vi "ODOR_BLASTER_V22.3 Final.vi"() -> ()   [LabVIEW 2022 SP3]
uses:
  <vilib>/Utility/error.llb/DialogType.ctl
  <vilib>/DAQmx/read.llb/DAQmx Read (Analog Wfm 1Chan NSamp).vi
  <vilib>/DAQmx/write.llb/DAQmx Write (Digital 1D Bool NChan 1Samp 1Line).vi
  <vilib>/gmath/statdist.llb/Random Permutation.vi
  <vilib>/DAQmx/create/channels.llb/DAQmx Create Channel (AI-Voltage-Basic).vi
  <vilib>/DAQmx/configure/timing.llb/DAQmx Timing (Sample Clock).vi
  <vilib>/DAQmx/miscellaneous.llb/DAQmx Fill In Error Info.vi
  <vilib>/Waveform/WDTOps.llb/WDT Append Waveforms DBL.vi
  <vilib>/Waveform/WDTFileIO.llb/Export Waveform To Spreadsheet File.vi
  <vilib>/gmath/NI_Gmath.lvlib
panel:
  out "Elapsed Time (s)":dbl
  out "source out 2":string
  out "error out 2":errorcluster
  out "Waveform Chart 2":waveform(dbl)(graph)
  out "source out":string
  out "error out":errorcluster
  out "RECORDING TIME (s)":dbl
  out "Waveform Chart":waveform(dbl)(graph)
  in  "How long recording lasts (s)":u32=4 caption="Time Target (s)"
  out "Device Running":bool
  in  "Time Between Loops (s)":i32=1
  in  "Presentation mode":u8(ring) items=["Sequential", "Random", "Simultaneous"]
  in  "Initial Delay (s)":u32=10
  out "Coming up next":bool[](array[boolean])
  in  "manual trigger":bool
  in  "Number of Puffs per trial":i32=1
  out "Puffing":bool
  in  "Puff Duration (s)":u32=2000
  in  "Valves to use":bool[](array[boolean])
  # "1"
  # "2"
  # "3"
  # "4"
  # "5"
  # "6"
  # "7"
  # "8"
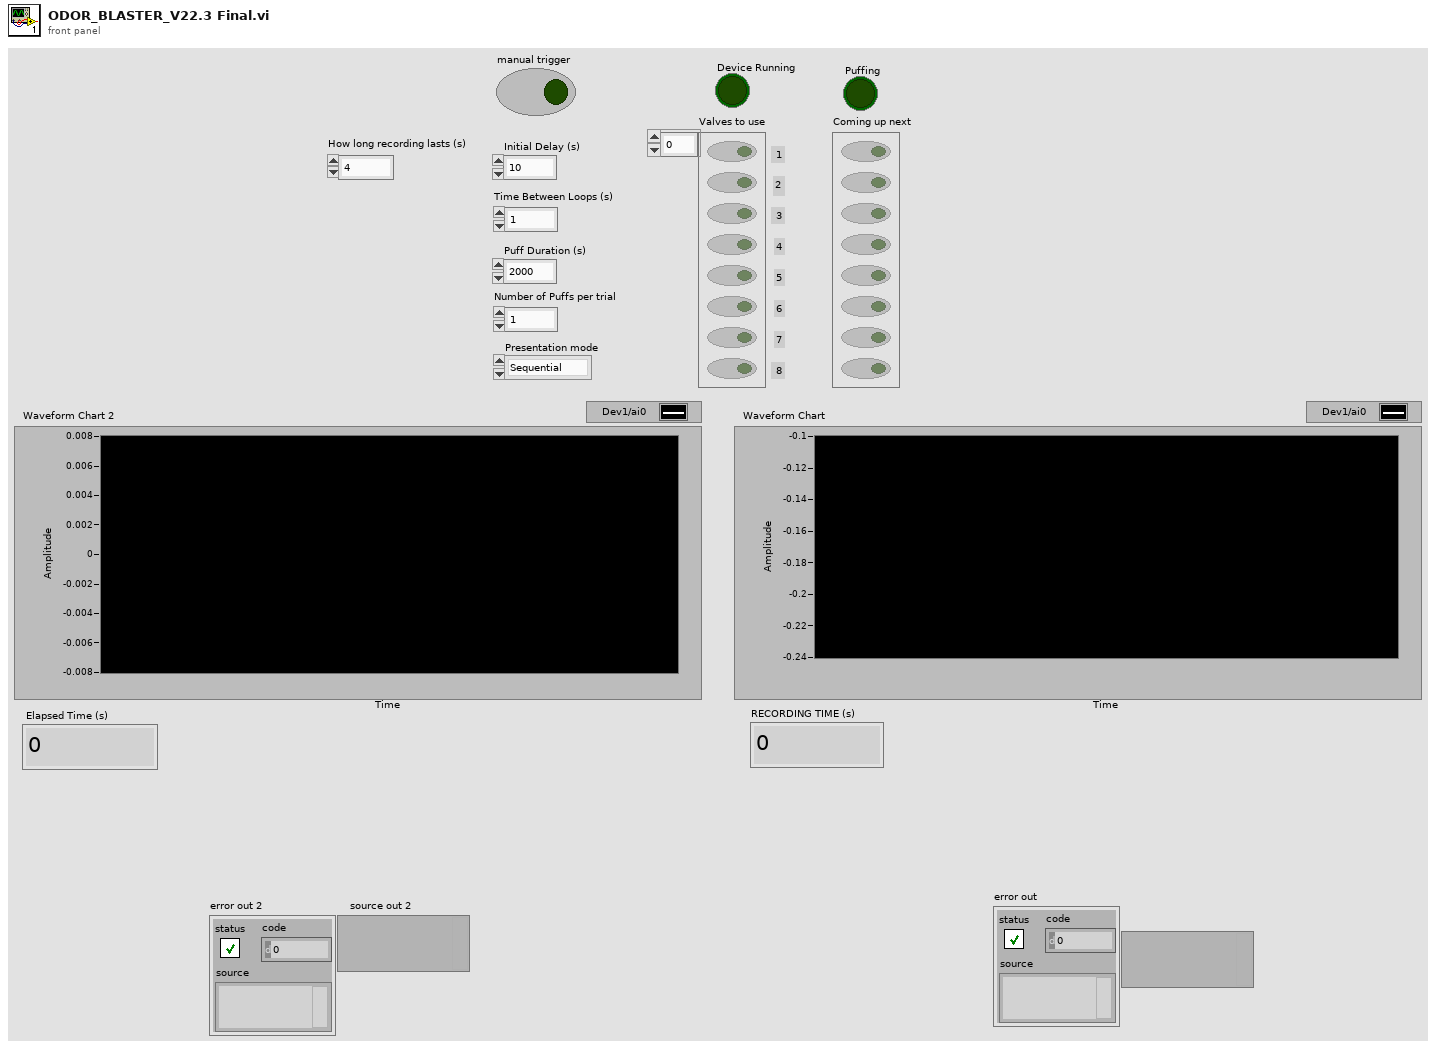
[diagram p1: front panel]
types:
  T1 = typedef "DialogType.ctl" = u16
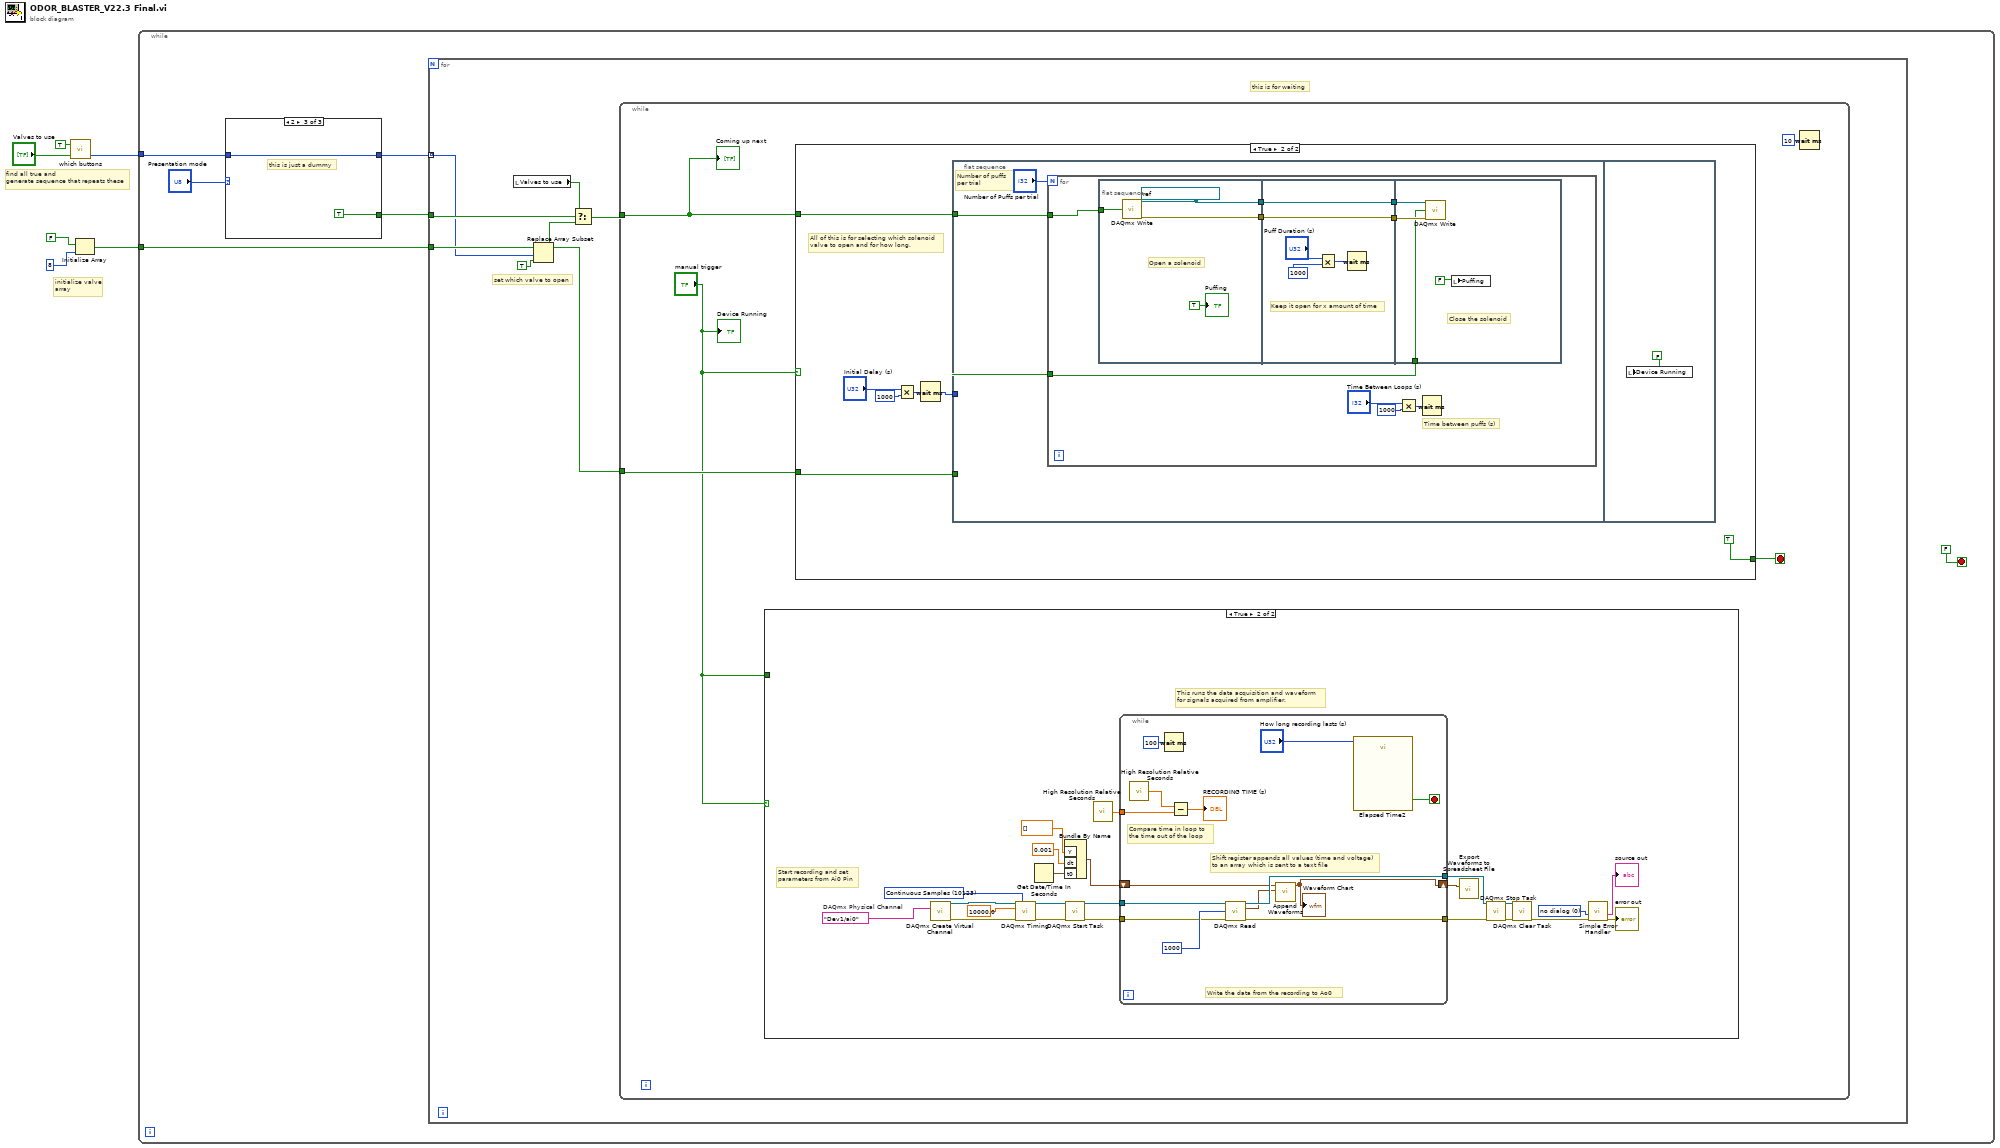
[diagram p0: block diagram]
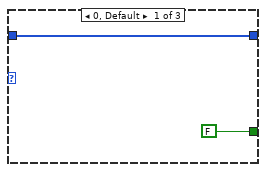
[diagram p2: hidden frame]
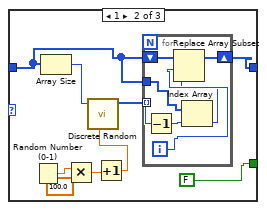
[diagram p3: hidden frame]
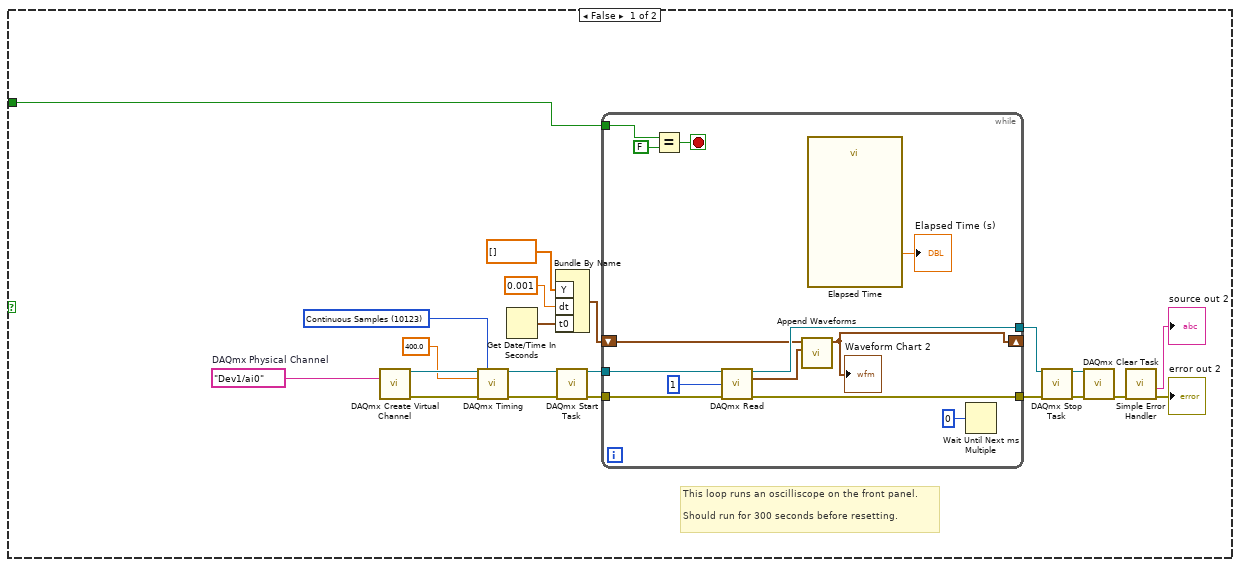
[diagram p4: hidden frame]
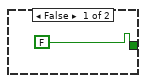
[diagram p5: hidden frame]
diagram:
  # "initialize valve\narray"
  # "find all true and\ngenerate sequence that repeats these"
  n1 = call "which buttons.vi"("boolean array"="Valves to use", "true/false"=TRUE) -> ("indexes of matching booleans"=w4:i32[])  [unwired: 1 in]
  n2 = Initialize Array(FALSE, 8 ("dimension size")) -> (w1:bool[])
  n3 = while {
    tunnel: w4 -> [w10]
    tunnel: w1 -> [w11]
    stop <- FALSE stop-if-true
    n4 = case shown="2" "Presentation mode" {
      tunnel: w10 -> [w14 w21 w32]
      tunnel: [w14 w20 w32] -> w7
      tunnel: [FALSE FALSE TRUE] -> w8
      frame 0, Default {
      }
      frame 1 {
        n5 = Random Number (0-1)() -> (number: 0 to 1=w19:dbl)
        n6 = Array Size(array=w21) -> (size(s)=w23:i32)
        n7 = Multiply(x=w19, y=100.0) -> (x*y=w17:dbl)
        n8 = Increment(x=w17) -> (x+1=w16:dbl)
        n9 = call-poly <vilib>:"Discrete Random.vi"("seed"=w16, "N"=w23) -> ("random permutation"=w22:i32[])  [unwired: 8 in, 1 out]
        n10 = for {
          tunnel: w22 -> [w30] mode=indexing
          shift-right: [w27] -> w20
          shift-left: w21 -> [w28]
          tunnel: w21 -> [w25]
          i -> [w26]
          n11 = Decrement(x=w30) -> (x-1=w29:i32)
          n12 = Index Array(array=w25, index=w29) -> (element=w24:i32)
          n13 = Replace Array Subset(array=w28, new element=w24, index=w26) -> (w27:i32[])
        }
      }
      frame 2 {
        # "this is just a dummy"
      }
    }
    n14 = for {
      tunnel: w11 -> [w37]
      tunnel: w8 -> [w38]
      tunnel: w7 -> [w33] mode=indexing
      # "set which valve to open"
      # "this is for waiting"
      n15 = local read "Valves to use"() -> (w36:bool[])
      n16 = Replace Array Subset(array=w37, new element=TRUE ("new element/subarray"), index=w33) -> (w35:bool[])
      n17 = Select(t=w36, s=w38, f=w35) -> (s? t:f=w34:bool[])
      n18 = while {
        tunnel: w34 -> [w43]
        tunnel: w37 -> [w42]
        stop <- w40 stop-if-true
        n19 = case shown="True" "manual trigger" {
          tunnel: "manual trigger" -> [w45 _]
          frame False {
            w50 = tag "Dev1/ai0"  # DAQmx Physical Channel
            w49 = 10123 items=["Finite Samples"=10178, "Continuous Samples"=10123, "Hardware Timed Single Point"=12522] ("sample mode")
            # "This loop runs an oscilliscope on the front panel.\n\nShould run for 300 seconds before resetting."
            n20 = call-poly <vilib>:"DAQmx Create Virtual Channel.vi"("physical channels"=w50) -> ("task out"=w52:refnum<k21>, "error out"=w51:errorcluster)  [unwired: 13 in]
            n21 = call-poly <vilib>:"DAQmx Timing.vi"("task/channels in"=w52, "sample mode"=w49, "rate"=400.0, "error in"=w51) -> ("task out"=w59:refnum<k21>, "error out"=w60:errorcluster)  [unwired: 10 in]
            n22 = Get Date/Time In Seconds() -> (seconds since 1Jan1904=w58:timestamp)
            n23 = Bundle By Name("Y"=dbl[] [], "dt"=0.001, "t0"=w58) -> (w57:waveform(dbl))  [unwired: 1 in]
            n24 = call <vilib>:"DAQmx Start Task.vi"("task/channels in"=w59, "error in"=w60) -> ("task out"=w61:refnum<k21>, "error out"=w62:errorcluster)  [unwired: 12 in]
            n25 = while {
              tunnel: [w78] -> w53
              tunnel: [w77] -> w54
              tunnel: w61 -> [w74]
              tunnel: w62 -> [w73]
              shift-right: [w70] -> _
              shift-left: w57 -> [w71]
              tunnel: w45 -> [w68]
              stop <- w67 stop-if-true
              n26 = Equal?(x=w68, y=FALSE) -> (x = y?=w67:bool)
              n27 = call-poly <vilib>:"DAQmx Read.vi"("task/channels in"=w74, "number of samples per channel"=1, "error in"=w73) -> ("task out"=w78:refnum<k21>, "data"=w72:waveform(dbl), "error out"=w77:errorcluster)  [unwired: 10 in]
              n28 = call-poly <vilib>:"Append Waveforms.vi"("waveform B"=w72, "waveform A"=w71) -> ("waveform out"=w70:waveform(dbl))  [unwired: 8 in, 1 out]
              "Waveform Chart 2" <- w70
              n29 = call "Elapsed Time"() -> ("Elapsed Time (s)"=→"Elapsed Time (s)":dbl)  [unwired: 12 in, 7 out]
              n30 = Wait Until Next ms Multiple(millisecond multiple=u32 0) -> ()  [unwired: 1 out]
            }
            n31 = call <vilib>:"DAQmx Stop Task.vi"("task/channels in"=w53, "error in"=w54) -> ("task out"=w55:refnum<k21>, "error out"=w56:errorcluster)  [unwired: 12 in]
            n32 = call <vilib>:"DAQmx Clear Task.vi"("task in"=w55, "error in"=w56) -> ("error out"=w63:errorcluster)  [unwired: 13 in]
            n33 = call <vilib>:"Simple Error Handler.vi"("error in (no error)"=w63) -> ("source out"=→"source out 2":string, "error out"=→"error out 2":errorcluster)  [unwired: 4 in, 3 out]
          }
          frame True {
            w81 = T1 0 items=["no dialog", "OK message", "continue or stop message", "OK message + warnings", "continue/stop + warnings"] ("type of dialog (OK msg:1)")
            w97 = tag "Dev1/ai0"  # DAQmx Physical Channel
            w99 = 10123 items=["Finite Samples"=10178, "Continuous Samples"=10123, "Hardware Timed Single Point"=12522] ("sample mode")
            # "Start recording and set \nparameters from Ai0 Pin"
            # "This runs the data acquisition and waveform \nfor signals acquired from amplifier."
            n34 = call-poly <vilib>:"DAQmx Create Virtual Channel.vi"("physical channels"=w97) -> ("task out"=w100:refnum<k21>, "error out"=w101:errorcluster)  [unwired: 13 in]
            n35 = call-poly <vilib>:"DAQmx Timing.vi"("task/channels in"=w100, "sample mode"=w99, "rate"=10000.0, "error in"=w101) -> ("task out"=w87:refnum<k21>, "error out"=w86:errorcluster)  [unwired: 10 in]
            n36 = Get Date/Time In Seconds() -> (seconds since 1Jan1904=w89:timestamp)
            n37 = Bundle By Name("Y"=dbl[] [], "dt"=0.001, "t0"=w89) -> (w90:waveform(dbl))  [unwired: 1 in]
            n38 = call <vilib>:"DAQmx Start Task.vi"("task/channels in"=w87, "error in"=w86) -> ("task out"=w85:refnum<k21>, "error out"=w84:errorcluster)  [unwired: 12 in]
            n39 = call <vilib>:"High Resolution Relative Seconds.vi"() -> ("relative seconds"=w83:dbl)
            n40 = while {
              tunnel: [w113] -> w96
              tunnel: [w112] -> w95
              tunnel: w85 -> [w104]
              tunnel: w84 -> [w110]
              shift-right: [w105] -> w92
              shift-left: w90 -> [w103]
              tunnel: w83 -> [w106]
              stop <- w114 stop-if-true
              # "Shift register appends all values (time and voltage)\nto an array which is sent to a text file"
              # "Write the data from the recording to Ao0"
              # "Compare time in loop to \nthe time out of the loop"
              n41 = call <vilib>:"High Resolution Relative Seconds.vi"() -> ("relative seconds"=w108:dbl)
              n42 = Wait (ms)(milliseconds to wait=u32 100) -> ()  [unwired: 1 out]
              n43 = Subtract(x=w108, y=w106) -> (x-y=→"RECORDING TIME (s)":dbl)
              n44 = call-poly <vilib>:"DAQmx Read.vi"("task/channels in"=w104, "number of samples per channel"=1000, "error in"=w110) -> ("task out"=w113:refnum<k21>, "data"=w109:waveform(dbl), "error out"=w112:errorcluster)  [unwired: 10 in]
              n45 = call-poly <vilib>:"Append Waveforms.vi"("waveform B"=w109, "waveform A"=w103) -> ("waveform out"=w105:waveform(dbl))  [unwired: 8 in, 1 out]
              "Waveform Chart" <- w105
              n46 = call "Elapsed Time2"("Time Target (s)"="How long recording lasts (s)") -> ("Time has Elapsed"=w114:bool)  [unwired: 11 in, 7 out]
            }
            n47 = call-poly <vilib>:"Export Waveforms to Spreadsheet File.vi"("waveform"=w92) -> ()  [unwired: 9 in, 2 out]
            n48 = call <vilib>:"DAQmx Stop Task.vi"("task/channels in"=w96, "error in"=w95) -> ("task out"=w94:refnum<k21>, "error out"=w93:errorcluster)  [unwired: 12 in]
            n49 = call <vilib>:"DAQmx Clear Task.vi"("task in"=w94, "error in"=w93) -> ("error out"=w82:errorcluster)  [unwired: 13 in]
            n50 = call <vilib>:"Simple Error Handler.vi"("type of dialog (OK msg:1)"=w81, "error in (no error)"=w82) -> ("source out"=→"source out":string, "error out"=→"error out":errorcluster)  [unwired: 3 in, 3 out]
          }
        }
        n51 = case shown="True" "manual trigger" {
          tunnel: w43 -> [_ w123]
          tunnel: [FALSE TRUE] -> w40
          tunnel: w42 -> [_ w121]
          frame False {
          }
          frame True {
            # "All of this is for selecting which solenoid\nvalve to open and for how long."
            n52 = Multiply(x="Initial Delay (s)", y=1000) -> (x*y=w120:u32)
            n53 = Wait (ms)(milliseconds to wait=w120) -> (millisecond timer value=w117:u32)
            n54 = flat-sequence {
              tunnel: w121 -> [w125]
              tunnel: w123 -> [w126]
              tunnel: w117 -> [_]
              frame #0 {
                # "Number of puffs\nper trial"
                n55 = for {
                  N: "Number of Puffs per trial" -> [_]
                  tunnel: w126 -> [w135]
                  tunnel: w125 -> [w134]
                  # "Time between puffs (s)"
                  n56 = flat-sequence {
                    tunnel: w135 -> [w139]
                    tunnel: [w138] -> w132
                    tunnel: [w136] -> w130
                    tunnel: [w143] -> w133
                    tunnel: w132 -> [w143]
                    tunnel: [w144] -> w131
                    tunnel: w130 -> [w144]
                    tunnel: w134 -> [w146]
                    tunnel: w133 -> [w147]
                    tunnel: w131 -> [w148]
                    frame #0 {
                      w136 = refnum<k21> "8 Channel Control" ("task/channels in")
                      # "Open a solenoid"
                      n57 = call-poly <vilib>:"DAQmx Write.vi"("task/channels in"=w136, "data"=w139) -> ("error out"=w138:errorcluster)  [unwired: 11 in, 2 out]
                      "Puffing" <- TRUE
                    }
                    frame #1 {
                      # "Keep it open for x amount of time"
                      n58 = Multiply(x="Puff Duration (s)", y=1000) -> (x*y=w140:u32)
                      n59 = Wait (ms)(milliseconds to wait=w140) -> ()  [unwired: 1 out]
                    }
                    frame #2 {
                      # "Close the solenoid"
                      n60 = call-poly <vilib>:"DAQmx Write.vi"("task/channels in"=w148, "data"=w146, "error in"=w147) -> ()  [unwired: 10 in, 3 out]
                      n61 = local write "Puffing"(FALSE ("Puff")) -> ()
                    }
                  }
                  n62 = Multiply(x="Time Between Loops (s)", y=1000) -> (x*y=w127:i32)
                  n63 = Wait (ms)(milliseconds to wait=w127) -> ()  [unwired: 1 out]
                }
              }
              frame #1 {
                n64 = local write "Device Running"(FALSE ("Puff")) -> ()
              }
            }
          }
        }
        n65 = Wait (ms)(milliseconds to wait=u32 10) -> ()  [unwired: 1 out]
        "Coming up next" <- w43
        "Device Running" <- "manual trigger"
      }
    }
  }
